vi "Define Parameter.vi"(8 "error in (no error)":errorcluster, 11 "Analyze SecondMomentum in":refnum<class "Analyze SecondMomentum.lvclass">) -> (0 "error out":errorcluster, 3 "Analyze SecondMomentum out":refnum<class "Analyze SecondMomentum.lvclass">)   [LabVIEW 2020, in "Analyze.lvlib" / "Analyze SecondMomentum.lvclass"]
uses:
  Analyze SecondMomentum.lvclass
  Analyze BaseClass/Analyze BaseClass/Analyze BaseClass.lvclass
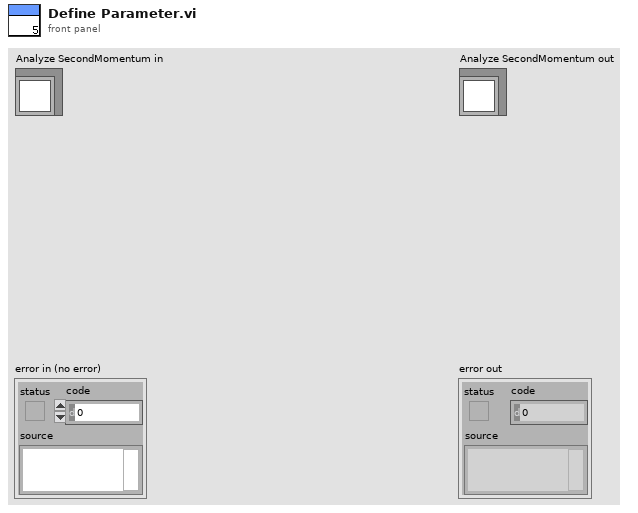
[diagram p1: front panel]
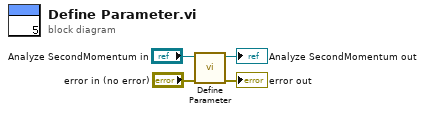
[diagram p0: block diagram]
diagram:
  n1 = call-parent "Define Parameter.vi"("error in (no error)"="error in (no error)", "Analyze BaseClass in"="Analyze SecondMomentum in") -> ("error out"=→"error out":errorcluster, "Analyze BaseClass out"=→"Analyze SecondMomentum out":refnum<class "Analyze SecondMomentum.lvclass">)  [unwired: 8 in]
